vi "Teardown.vi"(11 "Dev Actor Panel in":refnum<class "Dev Panel.lvclass">) -> (0 "error out":errorcluster)   [LabVIEW 2021, in "Dev Panel.lvclass"]
uses:
  Dev Panel.lvclass
  Dev Panel.lvclass/Dev Panel.ctl
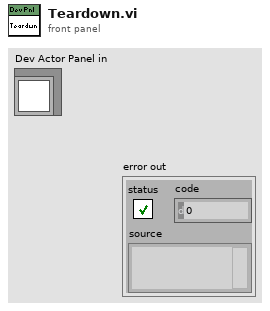
[diagram p1: front panel]
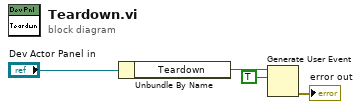
[diagram p0: block diagram]
diagram:
  n1 = Unbundle By Name("Dev Actor Panel in") -> ("Teardown"=w3:refnum<user-event>)
  n2 = Generate User Event(user event=w3, event data cluster=TRUE ("event data")) -> (error out=→"error out":errorcluster)  [unwired: 2 in, 1 out]
